vi "Read Variable Core.vi"(8 "error in":errorcluster, 10 "Variable Name":string, 11 "Spark Reference In":T1) -> (0 "error out":errorcluster, 2 "Variable Response":string, 3 "Spark Reference Out":T1)   [LabVIEW 2013, in "Spark API.lvlib"]
uses:
  Controls/Spark Reference.ctl
  <vilib>/httpClient/ClientHandle.ctl
  Controls/Device Query JSON.ctl
  Controls/Query Error JSON.ctl
  Spark API.lvlib
  <vilib>/httpClient/LabVIEWHTTPClient.lvlib
panel:
  out "body":string
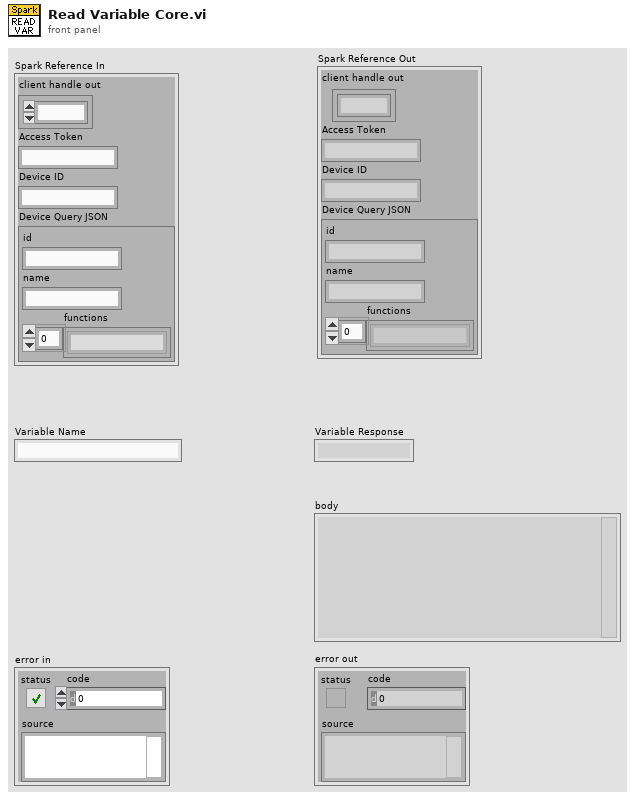
[diagram p1: front panel]
types:
  T1 = typedef "Spark API.lvlib/Spark Reference.ctl" = cluster{"client handle out":T2, "Access Token":string, "Device ID":string, "Device Query JSON":T3}
  T2 = typedef "LabVIEWHTTPClient.lvlib/ClientHandle.ctl" = refnum<k1>
  T3 = typedef "Spark API.lvlib/Device Query JSON.ctl" = cluster{"id":string, "name":string, "functions":string[]}
  T4 = typedef "Spark API.lvlib/Query Error JSON.ctl" = cluster{"code":dbl, "error":string, "error description":string}
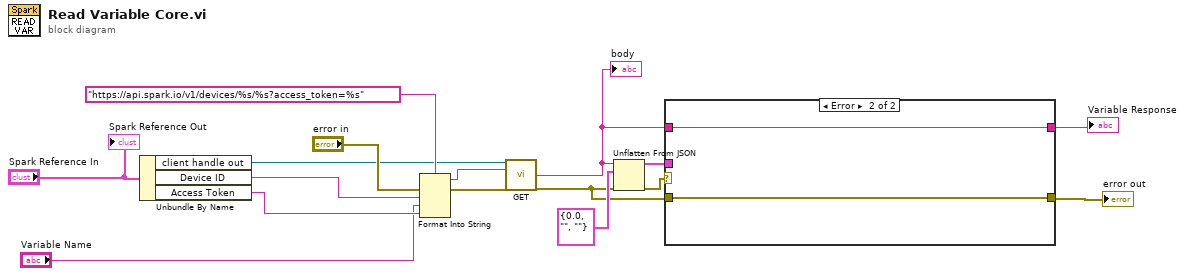
[diagram p0: block diagram]
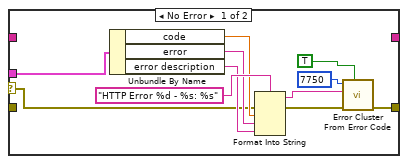
[diagram p2: hidden frame]
diagram:
  n1 = Unbundle By Name("Spark Reference In") -> ("client handle out"=w5:T2, "Device ID"=w4:string, "Access Token"=w3:string)
  n2 = Format Into String(format string="https://api.spark.io/v1/devices/%s/%s?access_token=%s" ("url"), error in="error in", w4, "Variable Name", w3) -> (resulting string=w15:string, error out=w6:errorcluster)  [unwired: 1 in]
  n3 = call <vilib>:"GET.vi"("client handle"=w5, "url"=w15, "error in (no error)"=w6) -> ("body"=w9:string, "error out"=w8:errorcluster)  [unwired: 9 in, 2 out]
  "body" <- w9
  n4 = Unflatten From JSON(JSON string=w9, type and defaults=T4 {"code"=0.0, "error"="", "error description"=""} ("Error JSON"), error in (no error)=w8) -> (value=w11:T4, error out=w12:errorcluster)  [unwired: 4 in]
  n5 = case shown="Error" w12 {
    selector: w12 -> [w18 _]
    tunnel: w11 -> [w27 _]
    tunnel: [w17 w29] -> w10
    tunnel: w9 -> [_ w28]
    tunnel: w8 -> [_ w29]
    tunnel: [_ w28] -> w1
    frame No Error {
      n6 = Unbundle By Name(w27) -> ("code"=w23:dbl, "error"=w22:string, "error description"=w21:string)
      n7 = Format Into String(format string="HTTP Error %d - %s: %s", error in=w18, w23, w22, w21) -> (resulting string=w20:string, error out=w19:errorcluster)  [unwired: 1 in]
      n8 = call <vilib>:"Error Cluster From Error Code.vi"("show call chain? (False)"=TRUE, "error in (no error)"=w19, "error message (\"\")"=w20, "error code (0)"=7750) -> ("error out"=w17:errorcluster)  [unwired: 5 in]
    }
    frame Error {
    }
  }
  "error out" <- w10
  "Variable Response" <- w1
  "Spark Reference Out" <- "Spark Reference In"
